vi "运维调试_五参数.vi"() -> ()   [LabVIEW 2016, in "斯坦道多参数.lvlib"]
uses:
  <vilib>/Utility/miscctls.llb/LVPointTypeDef.ctl
  <vilib>/Utility/config.llb/NI_LVConfig.lvlib
panel:
  in  "标样核查":bool
  in  "串口设置":bool
  in  "质控参数设置":bool
  in  "打开串口":bool
  in  "释放串口":bool
  out "多参数横条运行状态":T1(xcontrol)
  in  "数据区":i32(listbox)
  in  "停止测量(单探)":bool
  in  "启动测量(单探)":bool
  in  "控制命令区探头选择":u16(ring)=9 items=["氨氮"=3, "水温"=9, "pH值"=10, "溶解氧"=11, "电导率"=12, "浊度"=13, "叶绿素a"=14, "藻密度"=15, "蓝绿藻"=16, "氧化还原电位"=17, "溶解氧%"=18, "盐度"=19]
  in  "同步时间":bool
  in  "初始化(清洗)":bool
  in  "停止测量(全部)":bool
  in  "启动测量(全部)":bool
  in  "关键参数区读取":bool
  in  "关键参数区":i32(listbox)
  in  "传感器参数读取":bool
  in  "传感器区":i32(listbox)
  in  "返回":bool
  in  "设置":bool
  out "运行状态":string
  in  "停止":bool
  in  "水样测试":bool
  out "集成报警信息":string
  # "控制命令区"
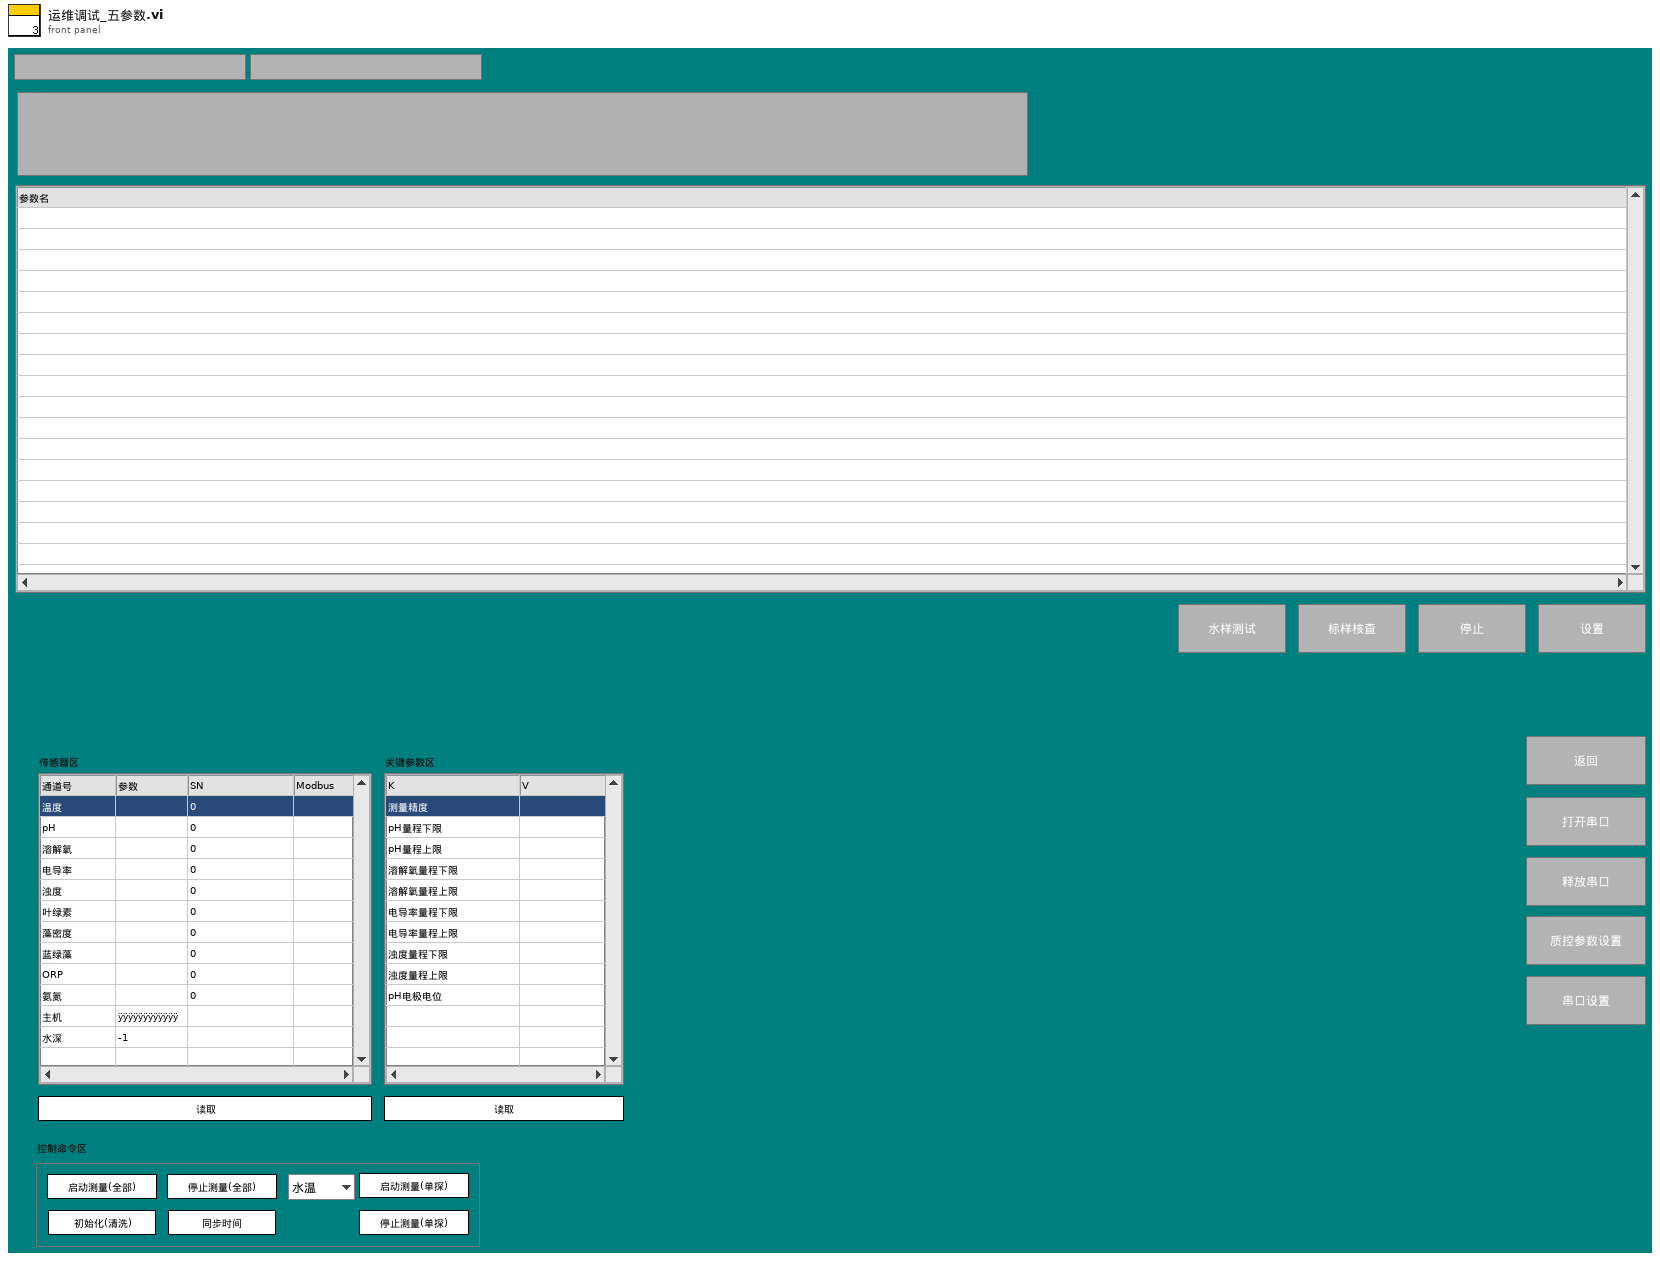
[diagram p1: front panel]
types:
  T1 = cluster{"系统时间":timestamp, "工作状态":u16, "测量模式":u16, "告警代码":enum16{"无告警", "缺试剂告警", "缺水样告警", "缺蒸馏水告警", "缺标液告警", "仪表漏液告警", "标定异常告警", "超量程告警", "加热异常", "低试剂预警", "超上限告警", "超下限告警", "仪表内部其他异常", "滴定异常告警", "电极异常告警", "量程切换告警", "参数设置告警", "PH电极电位异常", "电导率电极异常", "浊度光度异常", "溶解氧电极异常", "溶解氧光强异常", "温度异常告警", "PH异常告警", "溶解氧异常告警", "电导率异常告警", "浊度异常告警", "叶绿素异常告警", "藻密度异常告警", "蓝绿藻异常告警", "ORP异常告警", "氨氮异常告警", "清洁刷异常告警", "SD卡异常告警", "蓝牙异常告警", "Wifi异常告警", "流程异常告警"}, "故障代码":enum16{"无故障", "电机故障", "温度故障", "通讯故障", "滴定故障"}, "日志代码":u16, "软件版本":string}
  T2 = typedef "LVPointTypeDef.ctl" = cluster{"Horizontal":i16, "Vertical":i16}
  T3 = cluster{"时间标识":timestamp, "设备":string, "日志信息":string}
  T4 = enum16{"无告警", "缺试剂告警", "缺水样告警", "缺蒸馏水告警", "缺标液告警", "仪表漏液告警", "标定异常告警", "超量程告警", "加热异常", "低试剂预警", "超上限告警", "超下限告警", "仪表内部其他异常", "滴定异常告警", "电极异常告警", "量程切换告警", "参数设置告警", "PH电极电位异常", "电导率电极异常", "浊度光度异常", "溶解氧电极异常", "溶解氧光强异常", "温度异常告警", "PH异常告警", "溶解氧异常告警", "电导率异常告警", "浊度异常告警", "叶绿素异常告警", "藻密度异常告警", "蓝绿藻异常告警", "ORP异常告警", "氨氮异常告警", "清洁刷异常告警", "SD卡异常告警", "蓝牙异常告警", "Wifi异常告警", "流程异常告警"}
  T5 = cluster{"水温":dbl, "pH":dbl, "DO":dbl, "Cond":dbl, "Turb":dbl, "叶绿素":dbl, "藻密度":dbl, "蓝绿藻":dbl, "ORP":dbl, "NH3N":dbl}
  T6 = cluster{"因子编码":string, "单位":string, "标样参考值":sgl, "水样数据时间":timestamp, "水样实测值":sgl, "水样数据标识":string, "K":sgl, "B":sgl, "T":sgl, "H":sgl, "水深":sgl, "探头温度":sgl}
  T7 = typedef "NI_LVConfig.lvlib/Config Data RefNum.ctl" = refnum<k1>
  T8 = enum8{"Enabled", "Disabled", "Disabled and Grayed Out"}
  T9 = cluster{"测量模式":enum16{"待机", "水样测试", "标样核查", "零点核查", "跨度核查", "空白测试", "平行样测试", "加标回收", "空白校准", "标样校准", "初始化（清洗）"}, "数据标记表":string, "测量时间":dbl}
  T10 = cluster{"测量模式":enum16{"待机", "水样测试", "标样核查", "零点核查", "跨度核查", "空白测试", "平行样测试", "加标回收", "空白校准", "标样校准", "初始化（清洗）"}, "数据标记表":string, "输出参数":cluster{"水温":bool, "pH":bool, "DO":bool, "浊度":bool, "电导率":bool, "保存组数":dbl}}
  T11 = cluster{"水温标准液标准浓度":dbl, "酸碱度标准液标准浓度":dbl, "溶解氧标准液标准浓度":dbl, "电导率标准液标准浓度":dbl, "浊度标准液标准浓度":dbl}
  T12 = cluster{"确定":bool, "水温标准液标准浓度":dbl, "酸碱度标准液标准浓度":dbl, "溶解氧标准液标准浓度":dbl, "电导率标准液标准浓度":dbl, "浊度标准液标准浓度":dbl}
  T13 = enum32{"Bad", "Idle", "Run top level", "Running"}
  T14 = cluster{"水温":bool, "pH":bool, "DO":bool, "浊度":bool, "电导率":bool, "保存组数":dbl}
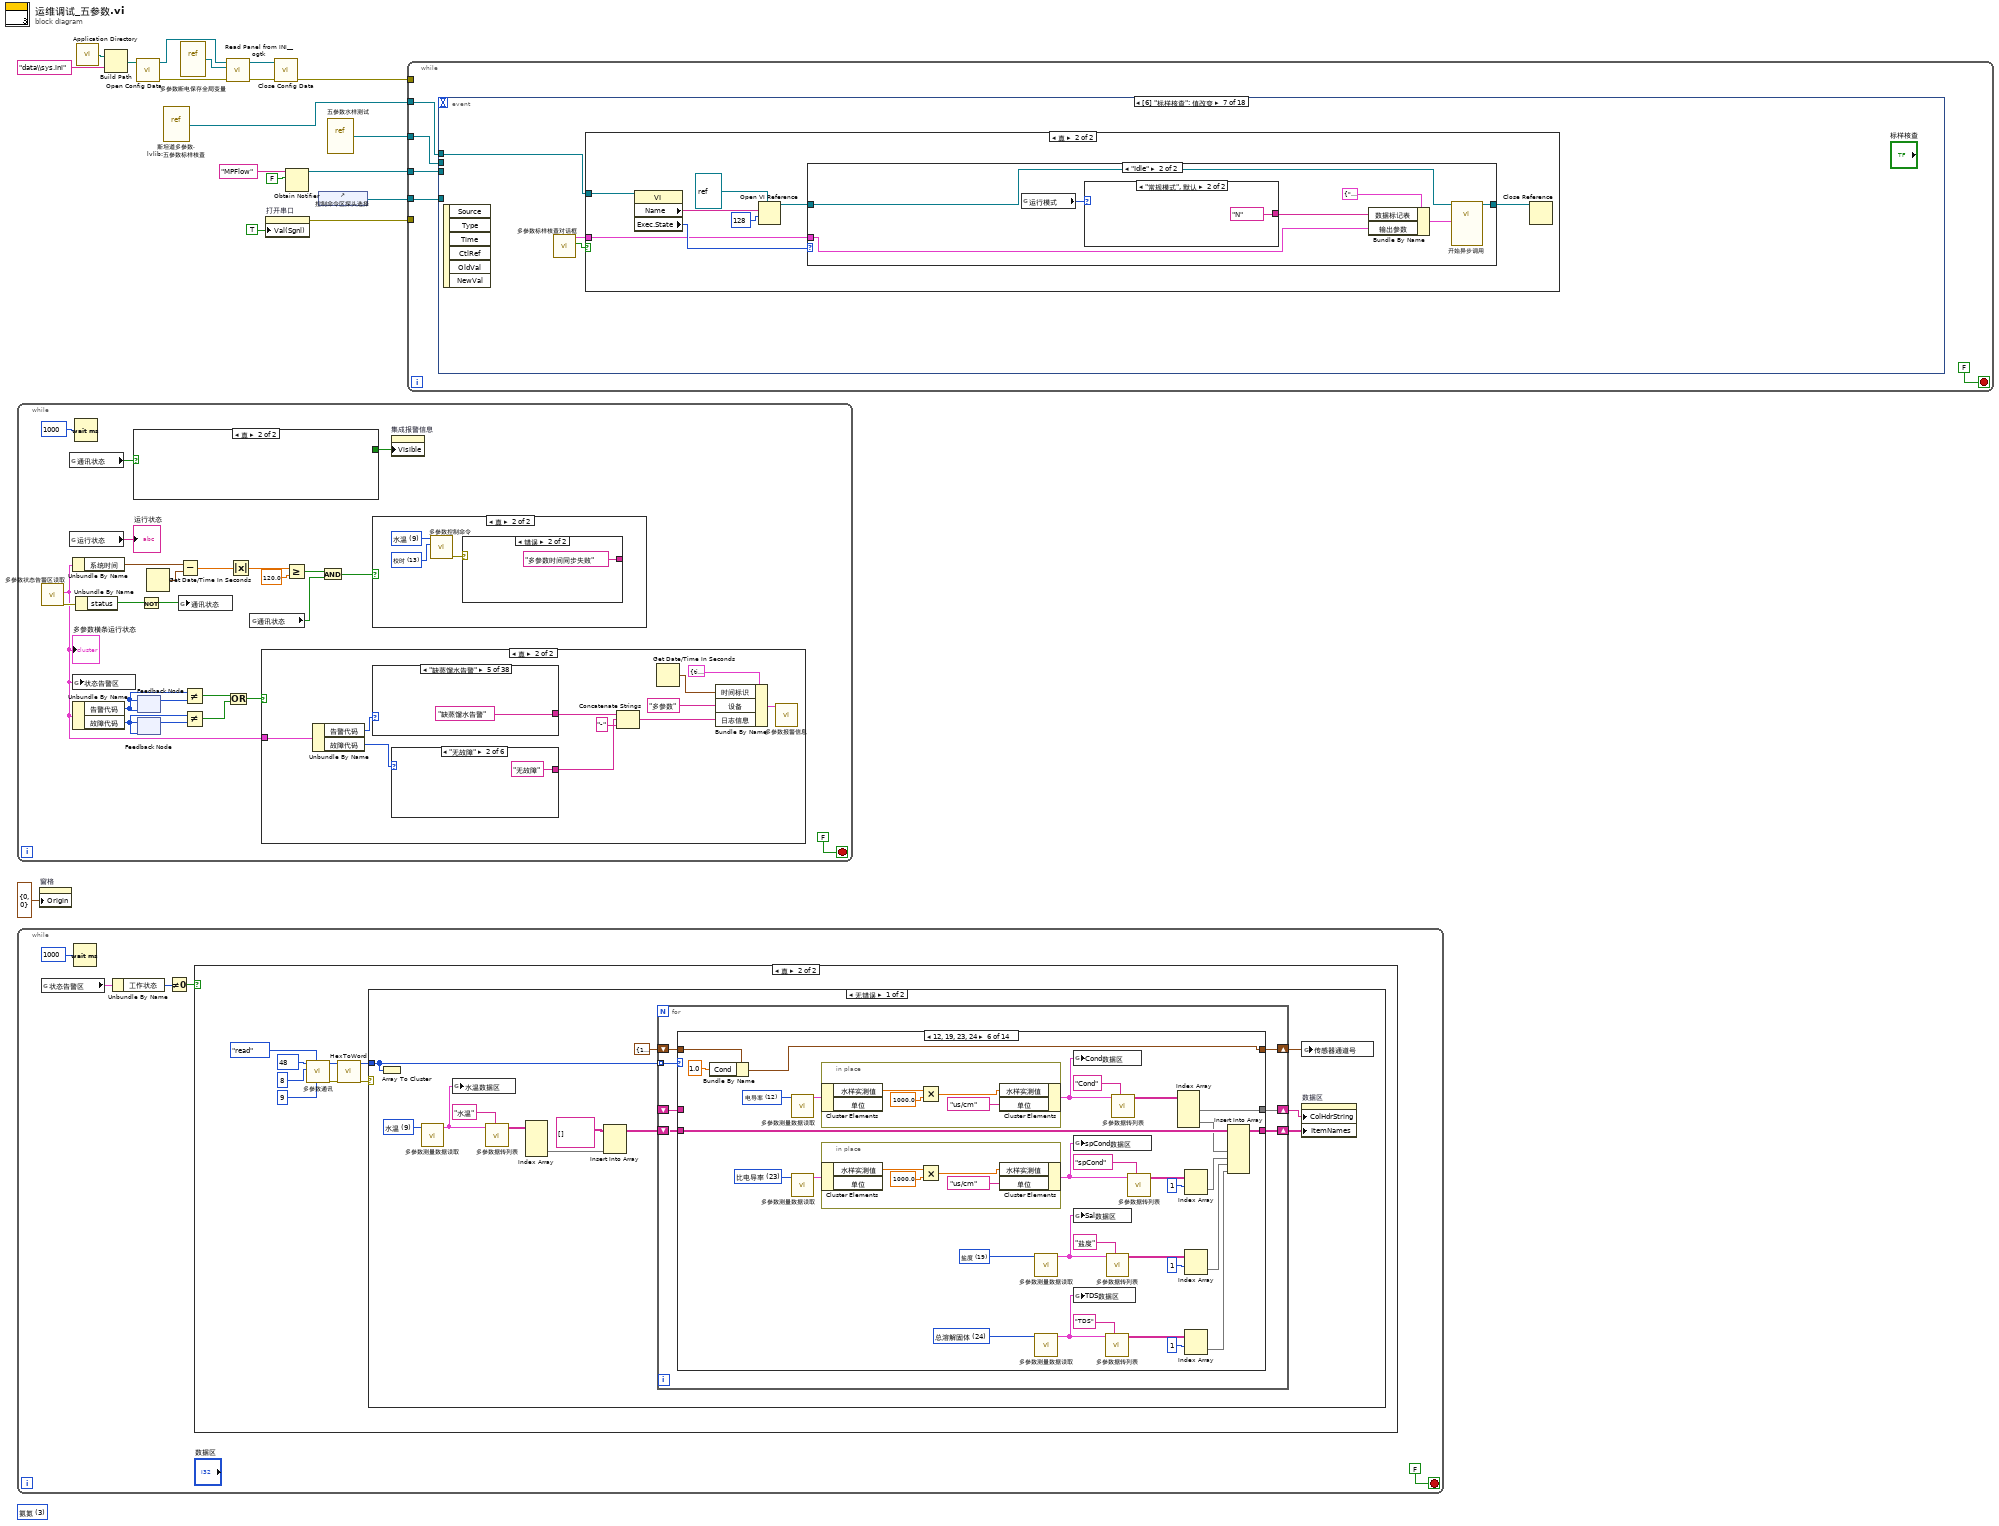
[diagram p0: block diagram]
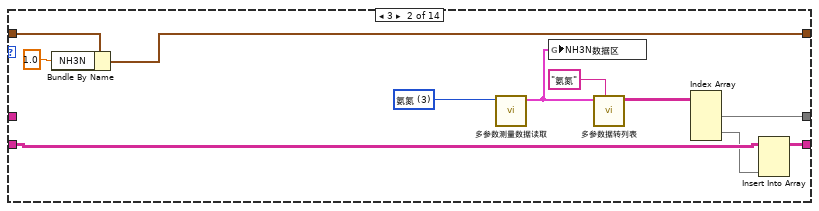
[diagram p4: hidden frame]
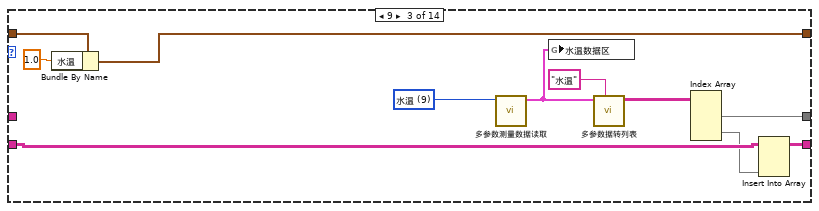
[diagram p5: hidden frame]
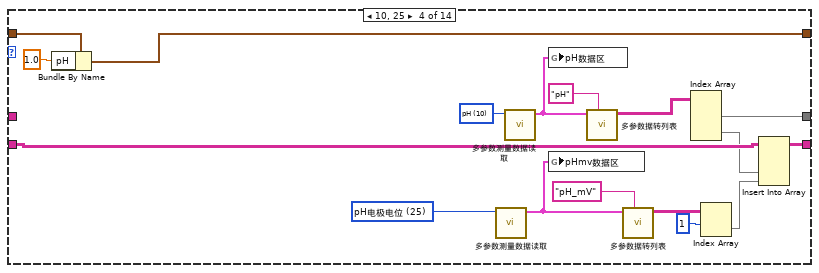
[diagram p6: hidden frame]
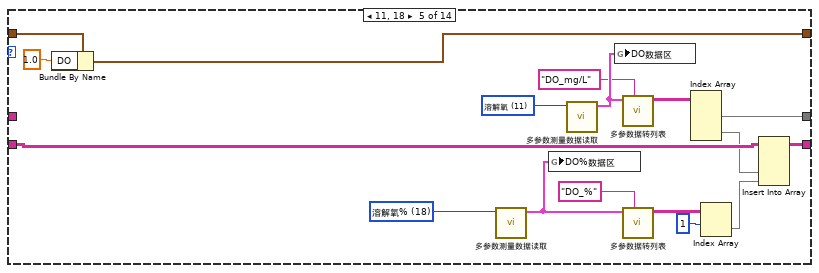
[diagram p7: hidden frame]
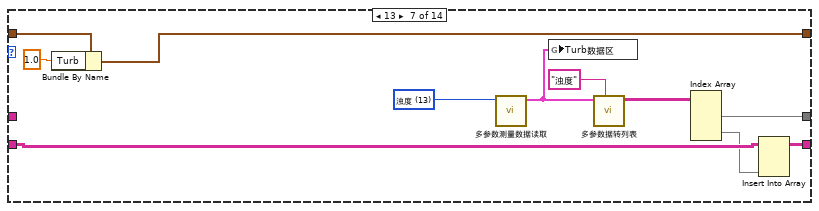
[diagram p8: hidden frame]
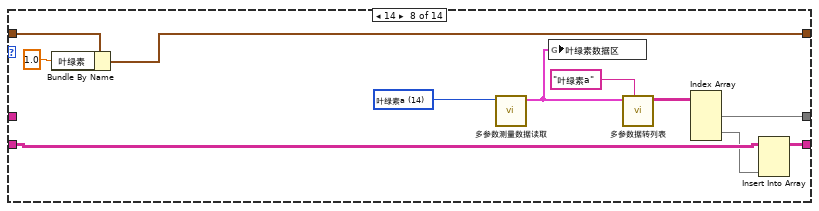
[diagram p9: hidden frame]
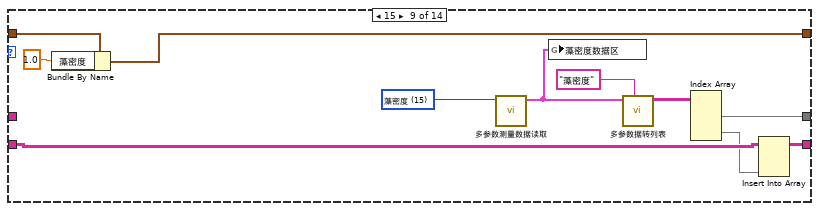
[diagram p10: hidden frame]
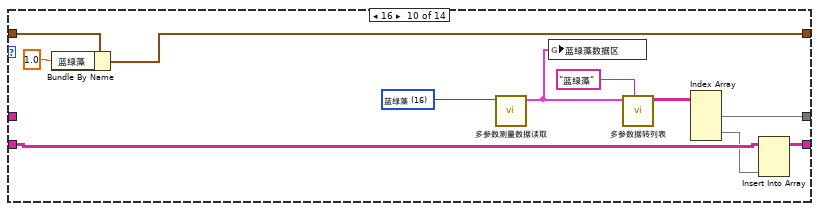
[diagram p11: hidden frame]
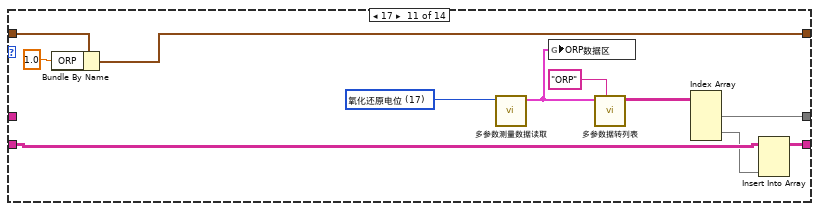
[diagram p12: hidden frame]
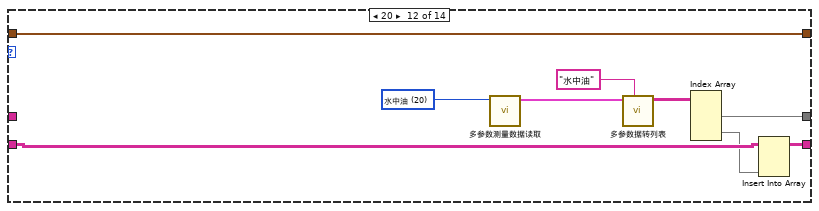
[diagram p13: hidden frame]
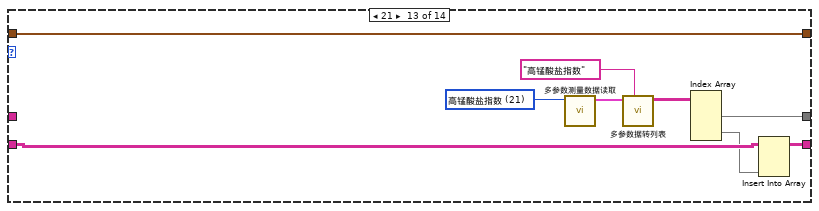
[diagram p14: hidden frame]
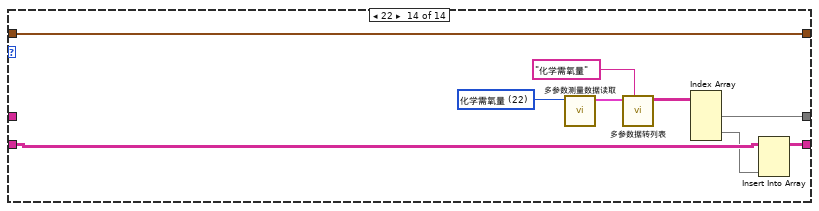
[diagram p15: hidden frame]
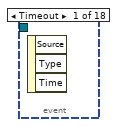
[diagram p17: hidden frame]
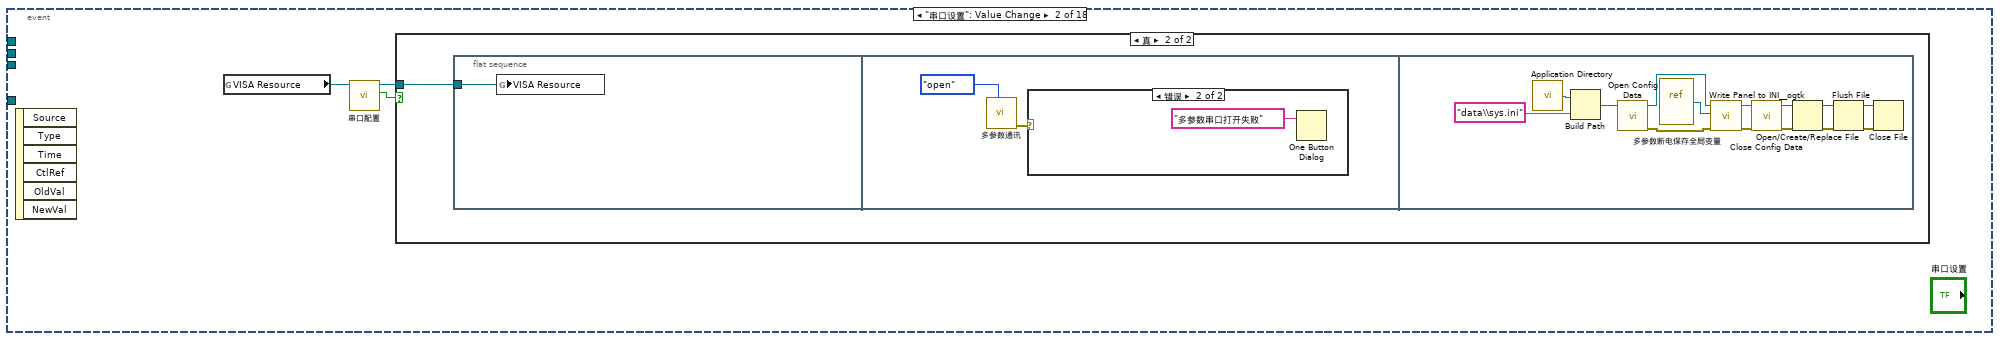
[diagram p18: hidden frame]
diagram:
  (unwired) u16 3 items=["氨氮"=3, "水温"=9, "pH"=10, "溶解氧"=11, "电导率"=12, "浊度"=13, "叶绿素a"=14, "藻密度"=15, "蓝绿藻"=16, "氧化还原电位"=17, "溶解氧%"=18, "盐度"=19, "水中油"=20, "高锰酸盐指数"=21, "化学需氧量"=22, "比电导率"=23, "总溶解固体"=24, "pH电极电位"=25] ("下拉列表")
  n1 = while {
    stop <- FALSE stop-if-true
    n2 = call "多参数状态告警区读取.vi"() -> ("error out"=w30:errorcluster, "状态告警块"=w27:T1)  [unwired: 9 in, 1 out]
    "多参数横条运行状态" <- w27
    n3 = global read "多参数全局变量.vi" "通讯状态"() -> (w40:bool)
    n4 = global read "多参数全局变量.vi" "运行状态"() -> (→"运行状态":string)
    n5 = Unbundle By Name(w27) -> ("系统时间"=w26:timestamp)
    n6 = global write "多参数全局变量.vi" "状态告警区"(w27) -> ()
    n7 = Unbundle By Name(w27) -> ("告警代码"=w36:T4, "故障代码"=w34:enum16{"无故障", "电机故障", "温度故障", "通讯故障", "滴定故障"})
    n8 = Wait (ms)(milliseconds to wait=u32 1000 ("等待时间（毫秒）")) -> ()  [unwired: 1 out]
    n9 = Unbundle By Name(w30) -> ("status"=w29:bool)
    n10 = case shown="真" w40 {
      tunnel: [TRUE ("可见") _] -> w39
      frame False {
        "集成报警信息" <- "通讯异常" ("集成报警信息")
      }
      frame True {
      }
    }
    n11 = feedback #1(w36) -> (w37:T4)
    n12 = feedback-in #1(w36) -> ()
    n13 = feedback #2(w34) -> (w35:enum16{"无故障", "电机故障", "温度故障", "通讯故障", "滴定故障"})
    n14 = feedback-in #2(w34) -> ()
    n15 = Not(x=w29) -> (.not. x?=w28:bool)
    n16 = Get Date/Time In Seconds() -> (seconds since 1Jan1904=w25:timestamp)
    n17 = Subtract(x=w26, y=w25) -> (x-y=w24:dbl)
    n18 = global write "多参数全局变量.vi" "通讯状态"(w28) -> ()
    n19 = Not Equal?(x=w36, y=w37) -> (x != y?=w32:bool)
    n20 = Not Equal?(x=w34, y=w35) -> (x != y?=w33:bool)
    n21 = Or(x=w32, y=w33) -> (x .or. y?=w31:bool)
    n22 = Absolute Value(x=w24) -> (abs(x)=w23:dbl)
    n23 = global read "多参数全局变量.vi" "通讯状态"() -> (w19:bool)
    n24 = case shown="真" w31 {
      tunnel: w27 -> [_ w58]
      frame False {
      }
      frame True {
        n25 = Unbundle By Name(w58) -> ("告警代码"=w57:T4, "故障代码"=w56:enum16{"无故障", "电机故障", "温度故障", "通讯故障", "滴定故障"})
        n26 = case shown="\"缺蒸馏水告警\"" w57 {
          selector: w57 -> [w69 _ _ _ _ _ _ _ _ _ _ _ _ _ _ _ _ _ _ _ _ _ _ _ _ _ _ _ _ _ _ _ _ _ _ _ _ _]
          tunnel: [w68 "无告警" "缺试剂告警" "缺水样告警" "缺蒸馏水告警" "缺标液告警" "仪表漏液告警" "标定异常告警" "超量程告警" "加热异常" "低试剂预警" "超上限告警" "超下限告警" "仪表内部其他异常" "滴定异常告警" "电极异常告警" "量程切换告警" "参数设置告警" "PH电极电位异常" "电导率电极异常" "浊度光度异常" "溶解氧电极异常" "溶解氧光强异常" "温度异常告警" "PH异常告警" "溶解氧异常告警" "电导率异常告警" "浊度异常告警" "叶绿素异常告警" "藻密度异常告警" "蓝绿藻异常告警" "ORP异常告警" "氨氮异常告警" "清洁刷异常告警" "SD卡异常告警" "蓝牙异常告警" "WiFi异常告警" "流程异常告警"] -> w55
          frame Default {
            n27 = Format Into String(format string="%d" ("格式字符串"), initial string="未知" ("工作状态"), w69) -> (resulting string=w68:string)  [unwired: 1 in, 1 out]
          }
          frame "无告警" {
          }
          frame "缺试剂告警" {
          }
          frame "缺水样告警" {
          }
          frame "缺蒸馏水告警" {
          }
          frame "缺标液告警" {
          }
          frame "仪表漏液告警" {
          }
          frame "标定异常告警" {
          }
          frame "超量程告警" {
          }
          frame "加热异常" {
          }
          frame "低试剂预警" {
          }
          frame "超上限告警" {
          }
          frame "超下限告警" {
          }
          frame "仪表内部其他异常" {
          }
          frame "滴定异常告警" {
          }
          frame "电极异常告警" {
          }
          frame "量程切换告警" {
          }
          frame "参数设置告警" {
          }
          frame "PH电极电位异常" {
          }
          frame "电导率电极异常" {
          }
          frame "浊度光度异常" {
          }
          frame "溶解氧电极异常" {
          }
          frame "溶解氧光强异常" {
          }
          frame "温度异常告警" {
          }
          frame "PH异常告警" {
          }
          frame "溶解氧异常告警" {
          }
          frame "电导率异常告警" {
          }
          frame "浊度异常告警" {
          }
          frame "叶绿素异常告警" {
          }
          frame "藻密度异常告警" {
          }
          frame "蓝绿藻异常告警" {
          }
          frame "ORP异常告警" {
          }
          frame "氨氮异常告警" {
          }
          frame "清洁刷异常告警" {
          }
          frame "SD卡异常告警" {
          }
          frame "蓝牙异常告警" {
          }
          frame "Wifi异常告警" {
          }
          frame "流程异常告警" {
          }
        }
        n28 = case shown="\"无故障\"" w56 {
          selector: w56 -> [w60 _ _ _ _ _]
          tunnel: [w59 "无故障" "电机故障" "温度故障" "通讯故障" "滴定故障"] -> w54
          frame Default {
            n29 = Format Into String(format string="%d" ("格式字符串"), initial string="未知" ("工作状态"), w60) -> (resulting string=w59:string)  [unwired: 1 in, 1 out]
          }
          frame "无故障" {
          }
          frame "电机故障" {
          }
          frame "温度故障" {
          }
          frame "通讯故障" {
          }
          frame "滴定故障" {
          }
        }
        n30 = Concatenate Strings(w55, "-" ("字符串"), w54) -> (w50:string)
        n31 = Get Date/Time In Seconds() -> (seconds since 1Jan1904=w49:timestamp)
        n32 = Bundle By Name(cluster=T3 {"时间标识"=timestamp(0 s since 1904-01-01), "设备"="", "日志信息"=""} ("data in"), "时间标识"=w49, "设备"="多参数", "日志信息"=w50) -> (w51:T3)
        n33 = call "多参数报警信息.vi"("data in"=w51) -> ()  [unwired: 10 in, 1 out]
      }
    }
    n34 = Greater Or Equal?(x=w23, y=120.0) -> (x >= y?=w22:bool)
    n35 = And(x=w22, y=w19) -> (x .and. y?=w20:bool)
    n36 = case shown="真" w20 {
      frame False {
      }
      frame True {
        w43 = u16 13 items=["启动测量（全部）"=1, "初始化（清洗）"=10, "停止测量（全部）"=11, "校时"=13, "启动测量（单个传感器）"=19, "停止测量（单个传感器）"=20] ("控制命令")
        w44 = u16 9 items=["氨氮"=3, "水温"=9, "pH值"=10, "溶解氧"=11, "电导率"=12, "浊度"=13, "叶绿素a"=14, "藻密度"=15, "蓝绿藻"=16, "氧化还原电位"=17, "溶解氧%"=18, "盐度"=19] ("站号")
        n37 = call "多参数控制命令.vi"("控制命令"=w43, "站号"=w44) -> ("error out"=w45:errorcluster)  [unwired: 9 in]
        n38 = case shown="错误" w45 {
          tunnel: ["多参数时间同步成功" ("消息") "多参数时间同步失败" ("消息")] -> _
          frame No Error {
          }
          frame Error {
          }
        }
      }
    }
    n39 = property on="集成报警信息" class="Str"("Visible"=w39) -> ()  [unwired: 2 in, 2 out]
  }
  n40 = while {
    stop <- FALSE stop-if-true
    n41 = global read "多参数全局变量.vi" "状态告警区"() -> (w113:T1)
    n42 = Wait (ms)(milliseconds to wait=u32 1000 ("等待时间（毫秒）")) -> ()  [unwired: 1 out]
    n43 = Unbundle By Name(w113) -> ("工作状态"=w112:u16)
    n44 = Not Equal To 0?(x=w112) -> (x != 0?=w111:bool)
    n45 = case shown="真" w111 {
      frame False {
      }
      frame True {
        n46 = call "多参数通讯.vi"("Slave ID"=u8 9, "STEP"=enum16{"open", "read", "write", "close"}."read", "quantity"=u16 8, "starting address"=u16 48) -> ("error out"=w118:errorcluster, "Registers"=w119:u16[])  [unwired: 5 in, 1 out]
        n47 = call "HexToWord.vi"("数组"=w119) -> ("WORD"=w122:u16[])  [unwired: 10 in]
        n48 = case shown="无错误" w118 {
          tunnel: w122 -> [w134 _]
          frame No Error {
            w131 = u16 9 items=["氨氮"=3, "水温"=9, "pH"=10, "溶解氧"=11, "电导率"=12, "浊度"=13, "叶绿素a"=14, "藻密度"=15, "蓝绿藻"=16, "氧化还原电位"=17, "溶解氧%"=18, "盐度"=19, "水中油"=20, "高锰酸盐指数"=21, "化学需氧量"=22, "比电导率"=23, "总溶解固体"=24, "pH电极电位"=25] ("下拉列表")
            n49 = Array To Cluster(array=w134) -> ()  [unwired: 1 out]
            n50 = call "多参数测量数据读取.vi"("探头选择"=w131) -> ("测量数据块"=w126:T6)  [unwired: 8 in, 2 out]
            n51 = global write "多参数全局变量.vi" "水温数据区"(w126) -> ()
            n52 = call "多参数据转列表.vi"("参数名"="水温", "测量数据块"=w126) -> ("添加的数组"=w124:string[][])  [unwired: 9 in]
            n53 = Index Array(array=w124) -> (element #2=w123:string[])  [unwired: 4 in, 1 out]
            n54 = Insert Into Array(array=string[][] [] ("子数组"), new element=w123) -> (w129:string[][])  [unwired: 2 in]
            n55 = for {
              tunnel: w134 -> [w141] mode=indexing
              shift-right: [w139] -> w132
              shift-left: w129 -> [w140]
              shift-right: [w138] -> w133
              shift-left: _ -> [w137]
              shift-right: [w136] -> w127
              shift-left: T5 {"水温"=1.0, "pH"=0.0, "DO"=0.0, "Cond"=0.0, "Turb"=0.0, "叶绿素"=0.0, "藻密度"=0.0, "蓝绿藻"=0.0, "ORP"=0.0, "NH3N"=0.0} ("传感器通道号") -> [w135]
              n56 = case shown="12, 19, 23, 24" w141 {
                tunnel: w140 -> [w144 w154 w165 w182 w199 w230 w249 w260 w271 w282 w293 w302 w311 w320]
                tunnel: [w144 w153 w164 w181 w198 w229 w248 w259 w270 w281 w292 w301 w310 w319] -> w139
                tunnel: [w143 w146 w157 w174 w191 w220 w242 w252 w265 w275 w286 w296 w305 w314] -> w138
                tunnel: w137 -> [w143 _ _ _ _ _ _ _ _ _ _ _ _ _]
                tunnel: [w142 w150 w161 w177 w195 w223 w245 w256 w267 w278 w289 w300 w309 w318] -> w136
                tunnel: w135 -> [w142 w152 w163 w179 w197 w224 w246 w257 w268 w279 w290 w300 w309 w318]
                frame 0, Default {
                }
                frame 3 {
                  w155 = u16 3 items=["氨氮"=3, "水温"=9, "pH"=10, "溶解氧"=11, "电导率"=12, "浊度"=13, "叶绿素a"=14, "藻密度"=15, "蓝绿藻"=16, "氧化还原电位"=17, "溶解氧%"=18, "盐度"=19, "水中油"=20, "高锰酸盐指数"=21, "化学需氧量"=22, "比电导率"=23, "总溶解固体"=24, "pH电极电位"=25] ("下拉列表")
                  n57 = Bundle By Name(cluster=w152, "NH3N"=1.0) -> (w150:T5)
                  n58 = call "多参数测量数据读取.vi"("探头选择"=w155) -> ("测量数据块"=w149:T6)  [unwired: 8 in, 2 out]
                  n59 = global write "多参数全局变量.vi" "NH3N数据区"(w149) -> ()
                  n60 = call "多参数据转列表.vi"("参数名"="氨氮", "测量数据块"=w149) -> ("添加的数组"=w148:string[][])  [unwired: 9 in]
                  n61 = Index Array(array=w148) -> (element #1=w146:string[], element #2=w145:string[])  [unwired: 4 in]
                  n62 = Insert Into Array(array=w154, new element=w145) -> (w153:string[][])  [unwired: 2 in]
                }
                frame 9 {
                  w166 = u16 9 items=["氨氮"=3, "水温"=9, "pH"=10, "溶解氧"=11, "电导率"=12, "浊度"=13, "叶绿素a"=14, "藻密度"=15, "蓝绿藻"=16, "氧化还原电位"=17, "溶解氧%"=18, "盐度"=19, "水中油"=20, "高锰酸盐指数"=21, "化学需氧量"=22, "比电导率"=23, "总溶解固体"=24, "pH电极电位"=25] ("下拉列表")
                  n63 = Bundle By Name(cluster=w163, "水温"=1.0) -> (w161:T5)
                  n64 = call "多参数测量数据读取.vi"("探头选择"=w166) -> ("测量数据块"=w160:T6)  [unwired: 8 in, 2 out]
                  n65 = global write "多参数全局变量.vi" "水温数据区"(w160) -> ()
                  n66 = call "多参数据转列表.vi"("参数名"="水温", "测量数据块"=w160) -> ("添加的数组"=w159:string[][])  [unwired: 9 in]
                  n67 = Index Array(array=w159) -> (element #1=w157:string[], element #2=w156:string[])  [unwired: 4 in]
                  n68 = Insert Into Array(array=w165, new element=w156) -> (w164:string[][])  [unwired: 2 in]
                }
                frame 10, 25 {
                  w180 = u16 25 items=["氨氮"=3, "水温"=9, "pH"=10, "溶解氧"=11, "电导率"=12, "浊度"=13, "叶绿素a"=14, "藻密度"=15, "蓝绿藻"=16, "氧化还原电位"=17, "溶解氧%"=18, "盐度"=19, "水中油"=20, "高锰酸盐指数"=21, "化学需氧量"=22, "比电导率"=23, "总溶解固体"=24, "pH电极电位"=25] ("下拉列表")
                  w183 = u16 10 items=["氨氮"=3, "水温"=9, "pH"=10, "溶解氧"=11, "电导率"=12, "浊度"=13, "叶绿素a"=14, "藻密度"=15, "蓝绿藻"=16, "氧化还原电位"=17, "溶解氧%"=18, "盐度"=19, "水中油"=20, "高锰酸盐指数"=21, "化学需氧量"=22, "比电导率"=23, "总溶解固体"=24, "pH电极电位"=25] ("下拉列表")
                  n69 = Bundle By Name(cluster=w179, "pH"=1.0) -> (w177:T5)
                  n70 = call "多参数测量数据读取.vi"("探头选择"=w180) -> ("测量数据块"=w170:T6)  [unwired: 8 in, 2 out]
                  n71 = call "多参数测量数据读取.vi"("探头选择"=w183) -> ("测量数据块"=w176:T6)  [unwired: 8 in, 2 out]
                  n72 = global write "多参数全局变量.vi" "pH数据区"(w176) -> ()
                  n73 = global write "多参数全局变量.vi" "pHmv数据区"(w170) -> ()
                  n74 = call "多参数据转列表.vi"("参数名"="pH", "测量数据块"=w176) -> ("添加的数组"=w175:string[][])  [unwired: 9 in]
                  n75 = call "多参数据转列表.vi"("参数名"="pH_mV", "测量数据块"=w170) -> ("添加的数组"=w169:string[][])  [unwired: 9 in]
                  n76 = Index Array(array=w175) -> (element #1=w174:string[], element #2=w173:string[])  [unwired: 4 in]
                  n77 = Index Array(array=w169, index (row)=1 ("禁用的索引 (列)")) -> (element=w172:string[])  [unwired: 1 in]
                  n78 = Insert Into Array(array=w182, new element #1=w173, new element #2=w172) -> (w181:string[][])  [unwired: 2 in]
                }
                frame 11, 18 {
                  w189 = u16 18 items=["氨氮"=3, "水温"=9, "pH"=10, "溶解氧"=11, "电导率"=12, "浊度"=13, "叶绿素a"=14, "藻密度"=15, "蓝绿藻"=16, "氧化还原电位"=17, "溶解氧%"=18, "盐度"=19, "水中油"=20, "高锰酸盐指数"=21, "化学需氧量"=22, "比电导率"=23, "总溶解固体"=24, "pH电极电位"=25] ("下拉列表")
                  w200 = u16 11 items=["氨氮"=3, "水温"=9, "pH"=10, "溶解氧"=11, "电导率"=12, "浊度"=13, "叶绿素a"=14, "藻密度"=15, "蓝绿藻"=16, "氧化还原电位"=17, "溶解氧%"=18, "盐度"=19, "水中油"=20, "高锰酸盐指数"=21, "化学需氧量"=22, "比电导率"=23, "总溶解固体"=24, "pH电极电位"=25] ("下拉列表")
                  n79 = Bundle By Name(cluster=w197, "DO"=1.0) -> (w195:T5)
                  n80 = call "多参数测量数据读取.vi"("探头选择"=w189) -> ("测量数据块"=w188:T6)  [unwired: 8 in, 2 out]
                  n81 = global write "多参数全局变量.vi" "DO%数据区"(w188) -> ()
                  n82 = call "多参数测量数据读取.vi"("探头选择"=w200) -> ("测量数据块"=w194:T6)  [unwired: 8 in, 2 out]
                  n83 = global write "多参数全局变量.vi" "DO数据区"(w194) -> ()
                  n84 = call "多参数据转列表.vi"("参数名"="DO_mg/L", "测量数据块"=w194) -> ("添加的数组"=w192:string[][])  [unwired: 9 in]
                  n85 = call "多参数据转列表.vi"("参数名"="DO_%", "测量数据块"=w188) -> ("添加的数组"=w186:string[][])  [unwired: 9 in]
                  n86 = Index Array(array=w192) -> (element #1=w191:string[], element #2=w190:string[])  [unwired: 4 in]
                  n87 = Index Array(array=w186, index (row)=1 ("禁用的索引 (列)")) -> (element=w185:string[])  [unwired: 1 in]
                  n88 = Insert Into Array(array=w199, new element #1=w190, new element #2=w185) -> (w198:string[][])  [unwired: 2 in]
                }
                frame 12, 19, 23, 24 {
                  w226 = u16 24 items=["氨氮"=3, "水温"=9, "pH"=10, "溶解氧"=11, "电导率"=12, "浊度"=13, "叶绿素a"=14, "藻密度"=15, "蓝绿藻"=16, "氧化还原电位"=17, "溶解氧%"=18, "盐度"=19, "水中油"=20, "高锰酸盐指数"=21, "化学需氧量"=22, "比电导率"=23, "总溶解固体"=24, "pH电极电位"=25] ("下拉列表")
                  w227 = u16 19 items=["氨氮"=3, "水温"=9, "pH"=10, "溶解氧"=11, "电导率"=12, "浊度"=13, "叶绿素a"=14, "藻密度"=15, "蓝绿藻"=16, "氧化还原电位"=17, "溶解氧%"=18, "盐度"=19, "水中油"=20, "高锰酸盐指数"=21, "化学需氧量"=22, "比电导率"=23, "总溶解固体"=24, "pH电极电位"=25] ("下拉列表")
                  w228 = u16 23 items=["氨氮"=3, "水温"=9, "pH"=10, "溶解氧"=11, "电导率"=12, "浊度"=13, "叶绿素a"=14, "藻密度"=15, "蓝绿藻"=16, "氧化还原电位"=17, "溶解氧%"=18, "盐度"=19, "水中油"=20, "高锰酸盐指数"=21, "化学需氧量"=22, "比电导率"=23, "总溶解固体"=24, "pH电极电位"=25] ("下拉列表")
                  w231 = u16 12 items=["氨氮"=3, "水温"=9, "pH"=10, "溶解氧"=11, "电导率"=12, "浊度"=13, "叶绿素a"=14, "藻密度"=15, "蓝绿藻"=16, "氧化还原电位"=17, "溶解氧%"=18, "盐度"=19, "水中油"=20, "高锰酸盐指数"=21, "化学需氧量"=22, "比电导率"=23, "总溶解固体"=24, "pH电极电位"=25] ("下拉列表")
                  n89 = Bundle By Name(cluster=w224, "Cond"=1.0 ("DO")) -> (w223:T5)
                  n90 = call "多参数测量数据读取.vi"("探头选择"=w231) -> ("测量数据块"=w207:T6)  [unwired: 8 in, 2 out]
                  n91 = call "多参数测量数据读取.vi"("探头选择"=w228) -> ("测量数据块"=w205:T6)  [unwired: 8 in, 2 out]
                  n92 = in-place {
                    n93 = in-place-cluster #3(w207) -> ("水样实测值"=w238:sgl)  [unwired: 1 out]
                    n94 = Multiply(x=w238, y=sgl 1000.0) -> (x*y=w236:sgl)
                    n95 = in-place-cluster #3("水样实测值"=w236, "单位"="us/cm") -> (w206:T6)
                  }
                  n96 = in-place {
                    n97 = in-place-cluster #4(w205) -> ("水样实测值"=w234:sgl)  [unwired: 1 out]
                    n98 = Multiply(x=w234, y=sgl 1000.0) -> (x*y=w232:sgl)
                    n99 = in-place-cluster #4("水样实测值"=w232, "单位"="us/cm") -> (w204:T6)
                  }
                  n100 = call "多参数测量数据读取.vi"("探头选择"=w227) -> ("测量数据块"=w214:T6)  [unwired: 8 in, 2 out]
                  n101 = call "多参数测量数据读取.vi"("探头选择"=w226) -> ("测量数据块"=w210:T6)  [unwired: 8 in, 2 out]
                  n102 = global write "多参数全局变量.vi" "Cond数据区"(w206) -> ()
                  n103 = global write "多参数全局变量.vi" "spCond数据区"(w204) -> ()
                  n104 = global write "多参数全局变量.vi" "Sal数据区"(w214) -> ()
                  n105 = global write "多参数全局变量.vi" "TDS数据区"(w210) -> ()
                  n106 = call "多参数据转列表.vi"("参数名"="TDS", "测量数据块"=w210) -> ("添加的数组"=w209:string[][])  [unwired: 9 in]
                  n107 = call "多参数据转列表.vi"("参数名"="盐度", "测量数据块"=w214) -> ("添加的数组"=w213:string[][])  [unwired: 9 in]
                  n108 = call "多参数据转列表.vi"("参数名"="Cond", "测量数据块"=w206) -> ("添加的数组"=w221:string[][])  [unwired: 9 in]
                  n109 = call "多参数据转列表.vi"("参数名"="spCond", "测量数据块"=w204) -> ("添加的数组"=w217:string[][])  [unwired: 9 in]
                  n110 = Index Array(array=w221) -> (element #1=w220:string[], element #2=w219:string[])  [unwired: 4 in]
                  n111 = Index Array(array=w217, index (row)=1 ("禁用的索引 (列)")) -> (element=w216:string[])  [unwired: 1 in]
                  n112 = Index Array(array=w213, index (row)=1 ("禁用的索引 (列)")) -> (element=w212:string[])  [unwired: 1 in]
                  n113 = Index Array(array=w209, index (row)=1 ("禁用的索引 (列)")) -> (element=w208:string[])  [unwired: 1 in]
                  n114 = Insert Into Array(array=w230, new element #1=w219, new element #2=w216, new element #3=w212, new element #4=w208) -> (w229:string[][])  [unwired: 2 in]
                }
                frame 13 {
                  w250 = u16 13 items=["氨氮"=3, "水温"=9, "pH"=10, "溶解氧"=11, "电导率"=12, "浊度"=13, "叶绿素a"=14, "藻密度"=15, "蓝绿藻"=16, "氧化还原电位"=17, "溶解氧%"=18, "盐度"=19, "水中油"=20, "高锰酸盐指数"=21, "化学需氧量"=22, "比电导率"=23, "总溶解固体"=24, "pH电极电位"=25] ("下拉列表")
                  n115 = Bundle By Name(cluster=w246, "Turb"=1.0 ("DO")) -> (w245:T5)
                  n116 = call "多参数测量数据读取.vi"("探头选择"=w250) -> ("测量数据块"=w240:T6)  [unwired: 8 in, 2 out]
                  n117 = global write "多参数全局变量.vi" "Turb数据区"(w240) -> ()
                  n118 = call "多参数据转列表.vi"("参数名"="浊度", "测量数据块"=w240) -> ("添加的数组"=w243:string[][])  [unwired: 9 in]
                  n119 = Index Array(array=w243) -> (element #1=w242:string[], element #2=w241:string[])  [unwired: 4 in]
                  n120 = Insert Into Array(array=w249, new element=w241) -> (w248:string[][])  [unwired: 2 in]
                }
                frame 14 {
                  w261 = u16 14 items=["氨氮"=3, "水温"=9, "pH"=10, "溶解氧"=11, "电导率"=12, "浊度"=13, "叶绿素a"=14, "藻密度"=15, "蓝绿藻"=16, "氧化还原电位"=17, "溶解氧%"=18, "盐度"=19, "水中油"=20, "高锰酸盐指数"=21, "化学需氧量"=22, "比电导率"=23, "总溶解固体"=24, "pH电极电位"=25] ("下拉列表")
                  n121 = Bundle By Name(cluster=w257, "叶绿素"=1.0 ("DO")) -> (w256:T5)
                  n122 = call "多参数测量数据读取.vi"("探头选择"=w261) -> ("测量数据块"=w255:T6)  [unwired: 8 in, 2 out]
                  n123 = global write "多参数全局变量.vi" "叶绿素数据区"(w255) -> ()
                  n124 = call "多参数据转列表.vi"("参数名"="叶绿素a", "测量数据块"=w255) -> ("添加的数组"=w253:string[][])  [unwired: 9 in]
                  n125 = Index Array(array=w253) -> (element #1=w252:string[], element #2=w251:string[])  [unwired: 4 in]
                  n126 = Insert Into Array(array=w260, new element=w251) -> (w259:string[][])  [unwired: 2 in]
                }
                frame 15 {
                  w272 = u16 15 items=["氨氮"=3, "水温"=9, "pH"=10, "溶解氧"=11, "电导率"=12, "浊度"=13, "叶绿素a"=14, "藻密度"=15, "蓝绿藻"=16, "氧化还原电位"=17, "溶解氧%"=18, "盐度"=19, "水中油"=20, "高锰酸盐指数"=21, "化学需氧量"=22, "比电导率"=23, "总溶解固体"=24, "pH电极电位"=25] ("下拉列表")
                  n127 = Bundle By Name(cluster=w268, "藻密度"=1.0 ("DO")) -> (w267:T5)
                  n128 = call "多参数测量数据读取.vi"("探头选择"=w272) -> ("测量数据块"=w264:T6)  [unwired: 8 in, 2 out]
                  n129 = global write "多参数全局变量.vi" "藻密度数据区"(w264) -> ()
                  n130 = call "多参数据转列表.vi"("参数名"="藻密度", "测量数据块"=w264) -> ("添加的数组"=w266:string[][])  [unwired: 9 in]
                  n131 = Index Array(array=w266) -> (element #1=w265:string[], element #2=w263:string[])  [unwired: 4 in]
                  n132 = Insert Into Array(array=w271, new element=w263) -> (w270:string[][])  [unwired: 2 in]
                }
                frame 16 {
                  w283 = u16 16 items=["氨氮"=3, "水温"=9, "pH"=10, "溶解氧"=11, "电导率"=12, "浊度"=13, "叶绿素a"=14, "藻密度"=15, "蓝绿藻"=16, "氧化还原电位"=17, "溶解氧%"=18, "盐度"=19, "水中油"=20, "高锰酸盐指数"=21, "化学需氧量"=22, "比电导率"=23, "总溶解固体"=24, "pH电极电位"=25] ("下拉列表")
                  n133 = Bundle By Name(cluster=w279, "蓝绿藻"=1.0 ("DO")) -> (w278:T5)
                  n134 = call "多参数测量数据读取.vi"("探头选择"=w283) -> ("测量数据块"=w277:T6)  [unwired: 8 in, 2 out]
                  n135 = global write "多参数全局变量.vi" "蓝绿藻数据区"(w277) -> ()
                  n136 = call "多参数据转列表.vi"("参数名"="蓝绿藻", "测量数据块"=w277) -> ("添加的数组"=w276:string[][])  [unwired: 9 in]
                  n137 = Index Array(array=w276) -> (element #1=w275:string[], element #2=w274:string[])  [unwired: 4 in]
                  n138 = Insert Into Array(array=w282, new element=w274) -> (w281:string[][])  [unwired: 2 in]
                }
                frame 17 {
                  w294 = u16 17 items=["氨氮"=3, "水温"=9, "pH"=10, "溶解氧"=11, "电导率"=12, "浊度"=13, "叶绿素a"=14, "藻密度"=15, "蓝绿藻"=16, "氧化还原电位"=17, "溶解氧%"=18, "盐度"=19, "水中油"=20, "高锰酸盐指数"=21, "化学需氧量"=22, "比电导率"=23, "总溶解固体"=24, "pH电极电位"=25] ("下拉列表")
                  n139 = Bundle By Name(cluster=w290, "ORP"=1.0 ("DO")) -> (w289:T5)
                  n140 = call "多参数测量数据读取.vi"("探头选择"=w294) -> ("测量数据块"=w288:T6)  [unwired: 8 in, 2 out]
                  n141 = global write "多参数全局变量.vi" "ORP数据区"(w288) -> ()
                  n142 = call "多参数据转列表.vi"("参数名"="ORP", "测量数据块"=w288) -> ("添加的数组"=w287:string[][])  [unwired: 9 in]
                  n143 = Index Array(array=w287) -> (element #1=w286:string[], element #2=w284:string[])  [unwired: 4 in]
                  n144 = Insert Into Array(array=w293, new element=w284) -> (w292:string[][])  [unwired: 2 in]
                }
                frame 20 {
                  w303 = u16 20 items=["氨氮"=3, "水温"=9, "pH"=10, "溶解氧"=11, "电导率"=12, "浊度"=13, "叶绿素a"=14, "藻密度"=15, "蓝绿藻"=16, "氧化还原电位"=17, "溶解氧%"=18, "盐度"=19, "水中油"=20, "高锰酸盐指数"=21, "化学需氧量"=22, "比电导率"=23, "总溶解固体"=24, "pH电极电位"=25] ("下拉列表")
                  n145 = call "多参数测量数据读取.vi"("探头选择"=w303) -> ("测量数据块"=w299:T6)  [unwired: 8 in, 2 out]
                  n146 = call "多参数据转列表.vi"("参数名"="水中油", "测量数据块"=w299) -> ("添加的数组"=w297:string[][])  [unwired: 9 in]
                  n147 = Index Array(array=w297) -> (element #1=w296:string[], element #2=w295:string[])  [unwired: 4 in]
                  n148 = Insert Into Array(array=w302, new element=w295) -> (w301:string[][])  [unwired: 2 in]
                }
                frame 21 {
                  w312 = u16 21 items=["氨氮"=3, "水温"=9, "pH"=10, "溶解氧"=11, "电导率"=12, "浊度"=13, "叶绿素a"=14, "藻密度"=15, "蓝绿藻"=16, "氧化还原电位"=17, "溶解氧%"=18, "盐度"=19, "水中油"=20, "高锰酸盐指数"=21, "化学需氧量"=22, "比电导率"=23, "总溶解固体"=24, "pH电极电位"=25] ("下拉列表")
                  n149 = call "多参数测量数据读取.vi"("探头选择"=w312) -> ("测量数据块"=w308:T6)  [unwired: 8 in, 2 out]
                  n150 = call "多参数据转列表.vi"("参数名"="高锰酸盐指数", "测量数据块"=w308) -> ("添加的数组"=w307:string[][])  [unwired: 9 in]
                  n151 = Index Array(array=w307) -> (element #1=w305:string[], element #2=w304:string[])  [unwired: 4 in]
                  n152 = Insert Into Array(array=w311, new element=w304) -> (w310:string[][])  [unwired: 2 in]
                }
                frame 22 {
                  w321 = u16 22 items=["氨氮"=3, "水温"=9, "pH"=10, "溶解氧"=11, "电导率"=12, "浊度"=13, "叶绿素a"=14, "藻密度"=15, "蓝绿藻"=16, "氧化还原电位"=17, "溶解氧%"=18, "盐度"=19, "水中油"=20, "高锰酸盐指数"=21, "化学需氧量"=22, "比电导率"=23, "总溶解固体"=24, "pH电极电位"=25] ("下拉列表")
                  n153 = call "多参数测量数据读取.vi"("探头选择"=w321) -> ("测量数据块"=w317:T6)  [unwired: 8 in, 2 out]
                  n154 = call "多参数据转列表.vi"("参数名"="化学需氧量", "测量数据块"=w317) -> ("添加的数组"=w316:string[][])  [unwired: 9 in]
                  n155 = Index Array(array=w316) -> (element #1=w314:string[], element #2=w313:string[])  [unwired: 4 in]
                  n156 = Insert Into Array(array=w320, new element=w313) -> (w319:string[][])  [unwired: 2 in]
                }
              }
            }
            n157 = global write "多参数全局变量.vi" "传感器通道号"(w127) -> ()
            n158 = property on="数据区" class="MCListbox (严格)"("ColHdrString"=w133, "ItemNames"=w132) -> ()  [unwired: 2 in, 2 out]
          }
          frame Error {
          }
        }
      }
    }
  }
  n159 = property on="窗格" class="Pane"("Origin"=T2 {"Horizontal"=0, "Vertical"=0} ("原点")) -> ()  [unwired: 2 in, 2 out]
  n160 = call <vilib>:"Application Directory.vi"() -> ("Application Directory"=w3:path)
  n161 = Build Path(base path=w3, name or relative path="data\\sys.ini" ("名称或相对路径")) -> (appended path=w5:path)
  n162 = call <vilib>:"Open Config Data.vi"("configuration file path"=w5) -> ("error out"=w9:errorcluster, "refnum"=w6:T7)  [unwired: 8 in, 1 out]
  n163 = vi-ref "斯坦道多参数.lvlib:五参数标样核查.vi"() -> (w1:refnum<vi>)
  n164 = vi-ref "多参数断电保存全局变量.vi"() -> (w7:refnum<vi>)
  n165 = call <userlib>:"Read Panel from INI__ogtk.vi"("error in (no error)"=w9, "VI ref"=w7, "refnum"=w6) -> ("error out"=w10:errorcluster, "refnum out"=w8:T7)  [unwired: 7 in]
  n166 = property on="打开串口" class="Bool (严格)"("Val(Sgnl)"=TRUE ("值(信号)")) -> (error out=w11:errorcluster)  [unwired: 2 in, 1 out]
  n167 = call <vilib>:"Close Config Data.vi"("error in (no error)"=w10, "refnum"=w8) -> ("error out"=w2:errorcluster)  [unwired: 8 in, 1 out]
  n168 = Obtain Notifier(name (unnamed)="MPFlow" ("名称（未命名）"), notification data type=FALSE) -> (notifier out=w14:refnum<notifier>)  [unwired: 2 in, 2 out]
  n169 = control-ref of="控制命令区探头选择"() -> (w13:refnum<vi>)
  n170 = vi-ref "五参数水样测试.vi"() -> (w15:refnum<vi>)
  n171 = while {
    tunnel: w15 -> [w325]
    tunnel: w14 -> [w324]
    tunnel: w13 -> [w323]
    tunnel: w11 -> [_]
    tunnel: w2 -> [_]
    tunnel: w1 -> [w322]
    stop <- FALSE stop-if-true
    n172 = event shown="[6] \"标样核查\": 值改变" {
      selector: _ -> [_ _ _ _ _ _ _ _ _ _ _ _ _ _ _ _ _ _]
      dyn-events: _ -> [_ _ _ _ _ _ _ _ _ _ _ _ _ _ _ _ _ _]
      timeout: _ -> [_ _ _ _ _ _ _ _ _ _ _ _ _ _ _ _ _ _]
      tunnel: w325 -> [_ _ _ _ _ w390 _ _ _ _ _ _ _ _ _ _ _ _]
      tunnel: w324 -> [_ _ _ _ _ _ _ w434 _ _ _ _ _ _ _ _ _ _]
      tunnel: w323 -> [_ _ _ _ _ _ _ _ _ _ _ _ _ _ _ _ w473 w480]
      tunnel: w322 -> [_ _ _ _ _ _ w411 _ _ _ _ _ _ _ _ _ _ _]
      event Timeout {
        n173 = event-data() -> ()  [unwired: 1 in, 3 out]
      }
      event "串口设置": Value Change {
        n174 = event-data() -> ()  [unwired: 1 in, 6 out]
        n175 = global read "多参数断电保存全局变量.vi" "VISA Resource"() -> (w329:refnum<visa-resource-name>)
        n176 = call "串口配置.vi"("VISA资源名称"=w329) -> ("确认 2"=w328:bool, "VISA资源名称 2"=w327:refnum<visa-resource-name>)  [unwired: 9 in]
        n177 = case shown="真" w328 {
          tunnel: w327 -> [_ w330]
          frame False {
          }
          frame True {
            n178 = flat-sequence {
              tunnel: w330 -> [w331]
              frame #0 {
                n179 = global write "多参数断电保存全局变量.vi" "VISA Resource"(w331) -> ()
              }
              frame #1 {
                n180 = call "多参数通讯.vi"("STEP"=enum16{"open", "read", "write", "close"}."open") -> ("error out"=w333:errorcluster)  [unwired: 8 in, 2 out]
                n181 = case shown="错误" w333 {
                  frame No Error {
                  }
                  frame Error {
                    n182 = One Button Dialog(message="多参数串口打开失败" ("消息")) -> ()  [unwired: 1 in, 1 out]
                  }
                }
              }
              frame #2 {
                n183 = call <vilib>:"Application Directory.vi"() -> ("Application Directory"=w348:path)
                n184 = Build Path(base path=w348, name or relative path="data\\sys.ini" ("名称或相对路径")) -> (appended path=w346:path)
                n185 = call <vilib>:"Open Config Data.vi"("configuration file path"=w346) -> ("error out"=w342:errorcluster, "refnum"=w345:T7)  [unwired: 8 in, 1 out]
                n186 = vi-ref "多参数断电保存全局变量.vi"() -> (w344:refnum<vi>)
                n187 = call <userlib>:"Write Panel to INI__ogtk.vi"("error in (no error)"=w342, "VI ref"=w344, "refnum"=w345) -> ("error out"=w341:errorcluster, "refnum out"=w343:T7)  [unwired: 7 in]
                n188 = call <vilib>:"Close Config Data.vi"("error in (no error)"=w341, "refnum"=w343) -> ("error out"=w336:errorcluster, "file path"=w335:path)  [unwired: 8 in]
                n189 = Open/Create/Replace File(file path (use dialog)=w335, error in=w336) -> (refnum out=w339:refnum<file>, error out=w340:errorcluster)  [unwired: 4 in, 1 out]
                n190 = Flush File(refnum=w339, error in=w340) -> (refnum out=w338:refnum<file>, error out=w337:errorcluster)
                n191 = Close File(refnum=w338, error in=w337) -> ()  [unwired: 2 out]
              }
            }
          }
        }
      }
      event "质控参数设置": Value Change {
        n192 = event-data() -> ()  [unwired: 1 in, 6 out]
        n193 = global read "多参数断电保存全局变量.vi" "质控参数设置"() -> (w349:T11)
        n194 = call "多参数质控参数设置.vi"("质控参数设置"=w349) -> ("输出簇"=w350:T12)  [unwired: 10 in]
        n195 = Unbundle By Name(w350) -> ("确定"=w351:bool)
        n196 = case shown="真" w351 {
          tunnel: w350 -> [_ w353]
          tunnel: w349 -> [_ w352]
          frame False {
          }
          frame True {
            n197 = flat-sequence {
              tunnel: w353 -> [w361]
              tunnel: w352 -> [w360]
              frame #0 {
                n198 = Unbundle By Name(w361) -> ("水温标准液标准浓度"=w359:dbl, "酸碱度标准液标准浓度"=w358:dbl, "溶解氧标准液标准浓度"=w357:dbl, "电导率标准液标准浓度"=w356:dbl, "浊度标准液标准浓度"=w355:dbl)
                n199 = Bundle By Name(cluster=w360, "水温标准液标准浓度"=w359, "酸碱度标准液标准浓度"=w358, "溶解氧标准液标准浓度"=w357, "电导率标准液标准浓度"=w356, "浊度标准液标准浓度"=w355) -> (w354:T11)
                n200 = global write "多参数断电保存全局变量.vi" "质控参数设置"(w354) -> ()
              }
              frame #1 {
                n201 = call <vilib>:"Application Directory.vi"() -> ("Application Directory"=w375:path)
                n202 = Build Path(base path=w375, name or relative path="data\\sys.ini" ("名称或相对路径")) -> (appended path=w373:path)
                n203 = call <vilib>:"Open Config Data.vi"("configuration file path"=w373) -> ("error out"=w369:errorcluster, "refnum"=w372:T7)  [unwired: 8 in, 1 out]
                n204 = vi-ref "多参数断电保存全局变量.vi"() -> (w371:refnum<vi>)
                n205 = call <userlib>:"Write Panel to INI__ogtk.vi"("error in (no error)"=w369, "VI ref"=w371, "refnum"=w372) -> ("error out"=w368:errorcluster, "refnum out"=w370:T7)  [unwired: 7 in]
                n206 = call <vilib>:"Close Config Data.vi"("error in (no error)"=w368, "refnum"=w370) -> ("error out"=w363:errorcluster, "file path"=w362:path)  [unwired: 8 in]
                n207 = Open/Create/Replace File(file path (use dialog)=w362, error in=w363) -> (refnum out=w366:refnum<file>, error out=w367:errorcluster)  [unwired: 4 in, 1 out]
                n208 = Flush File(refnum=w366, error in=w367) -> (refnum out=w365:refnum<file>, error out=w364:errorcluster)
                n209 = Close File(refnum=w365, error in=w364) -> ()  [unwired: 2 out]
              }
            }
          }
        }
      }
      event "释放串口": Value Change {
        n210 = event-data() -> ("NewVal"=w376:bool)  [unwired: 1 in, 5 out]
        n211 = case shown="真" w376 {
          frame False {
          }
          frame True {
            n212 = call "多参数通讯.vi"("STEP"=enum16{"open", "read", "write", "close"}."close") -> ("error out"=w377:errorcluster)  [unwired: 8 in, 2 out]
            n213 = case shown="无错误" w377 {
              frame No Error {
                n214 = property on="打开串口" class="Bool (严格)"("DisabledEnum"=T8."Enabled" ("禁用")) -> ()  [unwired: 2 in, 2 out]
              }
              frame Error {
              }
            }
          }
        }
      }
      event "打开串口": Value Change {
        n215 = event-data() -> ("NewVal"=w380:bool)  [unwired: 1 in, 5 out]
        n216 = case shown="真" w380 {
          frame False {
          }
          frame True {
            n217 = call "多参数通讯.vi"("STEP"=enum16{"open", "read", "write", "close"}."open") -> ("error out"=w381:errorcluster)  [unwired: 8 in, 2 out]
            n218 = case shown="错误" w381 {
              tunnel: [T8."Disabled and Grayed Out" ("禁用") T8."Enabled" ("禁用")] -> w383
              frame No Error {
              }
              frame Error {
                n219 = One Button Dialog(message="多参数串口打开失败" ("消息")) -> ()  [unwired: 1 in, 1 out]
              }
            }
            n220 = property on="打开串口" class="Bool (严格)"("DisabledEnum"=w383, "Value"=FALSE ("打开串口")) -> ()  [unwired: 2 in, 2 out]
          }
        }
      }
      event "水样测试": Value Change {
        n221 = event-data() -> ()  [unwired: 1 in, 6 out]
        n222 = call "多参数启动参数对话框.vi"() -> ("确认"=w389:bool, "测量时间"=w388:dbl)  [unwired: 10 in]
        n223 = case shown="真" w389 {
          tunnel: w390 -> [_ w392]
          tunnel: w388 -> [_ w391]
          frame False {
          }
          frame True {
            n224 = property class="VI"(reference=w392) -> ("Name"=w396:string, "Exec.State"=w394:T13)  [unwired: 1 in, 2 out]
            n225 = Open VI Reference(type specifier VI Refnum (for type only)=refnum<vi> refnum ("类型说明符VI引用句柄（仅用于类型）"), vi path=w396, options=128 ("选项")) -> (vi reference=w395:refnum<vi>)  [unwired: 3 in, 1 out]
            n226 = case shown="\"Idle\"" w394 {
              tunnel: w395 -> [w400 w407]
              tunnel: [w400 w406] -> w393
              tunnel: w391 -> [_ w402]
              frame "Bad", Default {
                n227 = One Button Dialog(message="仪器已经启动，无需重复启动" ("消息")) -> ()  [unwired: 1 in, 1 out]
              }
              frame "Idle" {
                n228 = global read "多参数全局变量.vi" "运行模式"() -> (w401:enum16{"维护模式", "常规模式", "应急模式", "质控模式"})
                n229 = case shown="\"常规模式\", 默认" w401 {
                  tunnel: ["M" ("数据标记表") "hd" ("数据标记表")] -> w403
                  frame "维护模式" {
                  }
                  frame "常规模式", Default {
                  }
                }
                n230 = Bundle By Name(cluster=T9 {"测量模式"=enum."水样测试", "数据标记表"="", "测量时间"=0.0} ("启动参数"), "数据标记表"=w403, "测量时间"=w402) -> (w404:T9)
                n231 = call-by-ref "开始异步调用"(reference=w407, "启动参数"=w404) -> (reference out=w406:refnum<vi>)  [unwired: 12 in, 1 out]
              }
            }
            n232 = Close Reference(reference=w393) -> ()  [unwired: 1 in, 1 out]
          }
        }
      }
      event "标样核查": Value Change {
        n233 = event-data() -> ()  [unwired: 1 in, 6 out]
        n234 = call "多参数标样核查对话框.vi"() -> ("确认"=w412:bool, "输出参数"=w410:T14)  [unwired: 10 in]
        n235 = case shown="真" w412 {
          tunnel: w411 -> [_ w415]
          tunnel: w410 -> [_ w413]
          frame False {
          }
          frame True {
            n236 = property class="VI"(reference=w415) -> ("Name"=w419:string, "Exec.State"=w417:T13)  [unwired: 1 in, 2 out]
            n237 = Open VI Reference(type specifier VI Refnum (for type only)=refnum<vi> refnum, vi path=w419, options=128 ("选项")) -> (vi reference=w418:refnum<vi>)  [unwired: 3 in, 1 out]
            n238 = case shown="\"Idle\"" w417 {
              tunnel: w418 -> [w422 w429]
              tunnel: [w422 w428] -> w416
              tunnel: w413 -> [_ w423]
              frame "Bad", Default {
                n239 = One Button Dialog(message="仪器已经启动，无需重复启动" ("消息")) -> ()  [unwired: 1 in, 1 out]
              }
              frame "Idle" {
                n240 = global read "多参数全局变量.vi" "运行模式"() -> (w427:enum16{"维护模式", "常规模式", "应急模式", "质控模式"})
                n241 = case shown="\"常规模式\", 默认" w427 {
                  tunnel: ["M" ("数据标记表") "N" ("数据标记表")] -> w425
                  frame "维护模式" {
                  }
                  frame "常规模式", Default {
                  }
                }
                n242 = Bundle By Name(cluster=T10 {"测量模式"=enum."标样核查", "数据标记表"="", "输出参数"={"水温"=FALSE, "pH"=FALSE, "DO"=FALSE, "浊度"=FALSE, "电导率"=FALSE, "保存组数"=0.0}} ("启动参数"), "数据标记表"=w425, "输出参数"=w423) -> (w424:T10)
                n243 = call-by-ref "开始异步调用"(reference=w429, "启动参数"=w424) -> (reference out=w428:refnum<vi>)  [unwired: 12 in, 1 out]
              }
            }
            n244 = Close Reference(reference=w416) -> ()  [unwired: 1 in, 1 out]
          }
        }
      }
      event "停止": Value Change {
        n245 = event-data() -> ()  [unwired: 1 in, 6 out]
        n246 = Two Button Dialog(message="请再一次确认是否停止测量" ("消息")) -> (T button?=w432:bool)  [unwired: 2 in]
        n247 = case shown="真" w432 {
          tunnel: w434 -> [_ w437]
          frame False {
          }
          frame True {
            w435 = u16 11 items=["启动测量（全部）"=1, "初始化（清洗）"=10, "停止测量（全部）"=11, "校时"=13, "启动测量（单个传感器）"=19, "停止测量（单个传感器）"=20] ("控制命令")
            w436 = u16 10 items=["氨氮"=3, "水温"=9, "pH值"=10, "溶解氧"=11, "电导率"=12, "浊度"=13, "叶绿素a"=14, "藻密度"=15, "蓝绿藻"=16, "氧化还原电位"=17, "溶解氧%"=18, "盐度"=19] ("站号")
            n248 = Send Notification(notification=TRUE ("通知"), notifier=w437) -> ()  [unwired: 1 in, 2 out]
            n249 = call "多参数控制命令.vi"("控制命令"=w435, "站号"=w436) -> ()  [unwired: 9 in, 1 out]
          }
        }
      }
      event "设置": Value Change {
        n250 = event-data() -> ()  [unwired: 1 in, 6 out]
        n251 = property on="窗格" class="Pane"("Origin"=T2 {"Horizontal"=0, "Vertical"=628} ("原点")) -> ()  [unwired: 2 in, 2 out]
      }
      event "返回": Value Change {
        n252 = event-data() -> ()  [unwired: 1 in, 6 out]
        n253 = property on="窗格" class="Pane"("Origin"=T2 {"Horizontal"=0, "Vertical"=0} ("原点")) -> ()  [unwired: 2 in, 2 out]
      }
      event "传感器参数读取": Value Change {
        n254 = event-data() -> ()  [unwired: 1 in, 6 out]
        n255 = call "多参数传感器参数读取.vi"() -> ("error out"=w441:errorcluster, "添加的数组"=w442:string[][])  [unwired: 10 in]
        n256 = call <vilib>:"General Error Handler.vi"("error in (no error)"=w441) -> ()  [unwired: 10 in, 5 out]
        n257 = property on="传感器区" class="MCListbox (严格)"("ItemNames"=w442) -> ()  [unwired: 2 in, 2 out]
      }
      event "关键参数区读取": Value Change {
        n258 = event-data() -> ()  [unwired: 1 in, 6 out]
        n259 = call "多参数关键参数读取.vi"() -> ("error out"=w443:errorcluster, "添加的数组"=w444:string[][])  [unwired: 10 in]
        n260 = call <vilib>:"General Error Handler.vi"("error in (no error)"=w443) -> ()  [unwired: 10 in, 5 out]
        n261 = property on="关键参数区" class="MCListbox (严格)"("ItemNames"=w444) -> ()  [unwired: 2 in, 2 out]
      }
      event "同步时间": Value Change {
        w445 = u16 13 items=["启动测量（全部）"=1, "初始化（清洗）"=10, "停止测量（全部）"=11, "校时"=13, "启动测量（单个传感器）"=19, "停止测量（单个传感器）"=20] ("控制命令")
        w446 = u16 9 items=["氨氮"=3, "水温"=9, "pH值"=10, "溶解氧"=11, "电导率"=12, "浊度"=13, "叶绿素a"=14, "藻密度"=15, "蓝绿藻"=16, "氧化还原电位"=17, "溶解氧%"=18, "盐度"=19] ("站号")
        n262 = event-data() -> ()  [unwired: 1 in, 6 out]
        n263 = call "多参数控制命令.vi"("控制命令"=w445, "站号"=w446) -> ("error out"=w448:errorcluster)  [unwired: 9 in]
        n264 = case shown="错误" w448 {
          tunnel: ["时间同步成功" ("消息") "时间同步失败" ("消息")] -> w447
          frame No Error {
          }
          frame Error {
          }
        }
        n265 = One Button Dialog(message=w447) -> ()  [unwired: 1 in, 1 out]
      }
      event "启动测量(全部)": Value Change {
        w451 = u16 1 items=["启动测量（全部）"=1, "初始化（清洗）"=10, "停止测量（全部）"=11, "校时"=13, "启动测量（单个传感器）"=19, "停止测量（单个传感器）"=20] ("控制命令")
        w452 = u16 9 items=["氨氮"=3, "水温"=9, "pH值"=10, "溶解氧"=11, "电导率"=12, "浊度"=13, "叶绿素a"=14, "藻密度"=15, "蓝绿藻"=16, "氧化还原电位"=17, "溶解氧%"=18, "盐度"=19] ("站号")
        n266 = event-data() -> ()  [unwired: 1 in, 6 out]
        n267 = call "多参数控制命令.vi"("控制命令"=w451, "站号"=w452) -> ("error out"=w454:errorcluster)  [unwired: 9 in]
        n268 = case shown="无错误" w454 {
          tunnel: ["启动成功" ("消息") "启动失败" ("消息")] -> w453
          frame No Error {
          }
          frame Error {
          }
        }
        n269 = One Button Dialog(message=w453) -> ()  [unwired: 1 in, 1 out]
      }
      event "停止测量(全部)": Value Change {
        w459 = u16 11 items=["启动测量（全部）"=1, "初始化（清洗）"=10, "停止测量（全部）"=11, "校时"=13, "启动测量（单个传感器）"=19, "停止测量（单个传感器）"=20] ("控制命令")
        w460 = u16 9 items=["氨氮"=3, "水温"=9, "pH值"=10, "溶解氧"=11, "电导率"=12, "浊度"=13, "叶绿素a"=14, "藻密度"=15, "蓝绿藻"=16, "氧化还原电位"=17, "溶解氧%"=18, "盐度"=19] ("站号")
        n270 = event-data() -> ()  [unwired: 1 in, 6 out]
        n271 = call "多参数控制命令.vi"("控制命令"=w459, "站号"=w460) -> ("error out"=w458:errorcluster)  [unwired: 9 in]
        n272 = case shown="错误" w458 {
          tunnel: ["停止成功" ("消息") "停止失败" ("消息")] -> w457
          frame No Error {
          }
          frame Error {
          }
        }
        n273 = One Button Dialog(message=w457) -> ()  [unwired: 1 in, 1 out]
      }
      event "初始化(清洗)": Value Change {
        w465 = u16 10 items=["启动测量（全部）"=1, "初始化（清洗）"=10, "停止测量（全部）"=11, "校时"=13, "启动测量（单个传感器）"=19, "停止测量（单个传感器）"=20] ("控制命令")
        w466 = u16 9 items=["氨氮"=3, "水温"=9, "pH值"=10, "溶解氧"=11, "电导率"=12, "浊度"=13, "叶绿素a"=14, "藻密度"=15, "蓝绿藻"=16, "氧化还原电位"=17, "溶解氧%"=18, "盐度"=19] ("站号")
        n274 = event-data() -> ()  [unwired: 1 in, 6 out]
        n275 = call "多参数控制命令.vi"("控制命令"=w465, "站号"=w466) -> ("error out"=w463:errorcluster)  [unwired: 9 in]
        n276 = case shown="错误" w463 {
          tunnel: ["初始化成功" ("消息") "初始化失败" ("消息")] -> w464
          frame No Error {
          }
          frame Error {
          }
        }
        n277 = One Button Dialog(message=w464) -> ()  [unwired: 1 in, 1 out]
      }
      event "启动测量(单探)": Value Change {
        w469 = u16 19 items=["启动测量（全部）"=1, "初始化（清洗）"=10, "停止测量（全部）"=11, "校时"=13, "启动测量（单个传感器）"=19, "停止测量（单个传感器）"=20] ("控制命令")
        n278 = event-data() -> ()  [unwired: 1 in, 6 out]
        n279 = property class="Ring (严格)"(reference=w473) -> ("Value"=w472:u16)  [unwired: 1 in, 2 out]
        n280 = call "多参数控制命令.vi"("控制命令"=w469, "站号"=w472) -> ("error out"=w471:errorcluster)  [unwired: 9 in]
        n281 = case shown="无错误" w471 {
          tunnel: ["启动成功" ("消息") "启动失败" ("消息")] -> w470
          frame No Error {
          }
          frame Error {
          }
        }
        n282 = One Button Dialog(message=w470) -> ()  [unwired: 1 in, 1 out]
      }
      event "停止测量(单探)": Value Change {
        w476 = u16 20 items=["启动测量（全部）"=1, "初始化（清洗）"=10, "停止测量（全部）"=11, "校时"=13, "启动测量（单个传感器）"=19, "停止测量（单个传感器）"=20] ("控制命令")
        n283 = event-data() -> ()  [unwired: 1 in, 6 out]
        n284 = property class="Ring (严格)"(reference=w480) -> ("Value"=w479:u16)  [unwired: 1 in, 2 out]
        n285 = call "多参数控制命令.vi"("控制命令"=w476, "站号"=w479) -> ("error out"=w478:errorcluster)  [unwired: 9 in]
        n286 = case shown="错误" w478 {
          tunnel: ["停止成功" ("消息") "停止失败" ("消息")] -> w477
          frame No Error {
          }
          frame Error {
          }
        }
        n287 = One Button Dialog(message=w477) -> ()  [unwired: 1 in, 1 out]
      }
    }
  }
